vi "test_libssh2_channel_handle_extended_data2.vi"() -> ()   [LabVIEW 2013, in "libssh2_integration_tests.lvlib"]
uses:
  libssh2_integration_tests.lvlib
  <vilib>/addons/_JKI Toolkits/Caraya/classes/Test/Test.lvclass
  support/support.lvlib
  libssh2/libssh2.lvlib
  <vilib>/addons/_JKI Toolkits/Caraya/classes/Assert/Assert.lvclass
panel:
  out "error out":errorcluster
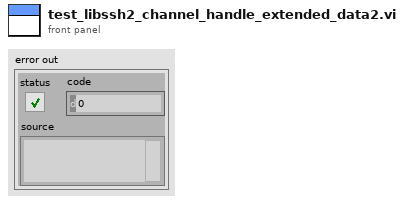
[diagram p1: front panel]
types:
  T1 = cluster{"mode":i32, "stdin":string, "stdout":string, "stderr":string}[]
  T2 = typedef "libssh2.lvlib/Session Refnum.ctl" = refnum<k1>
  T3 = typedef "libssh2.lvlib/Channel Refnum.ctl" = refnum<k1>
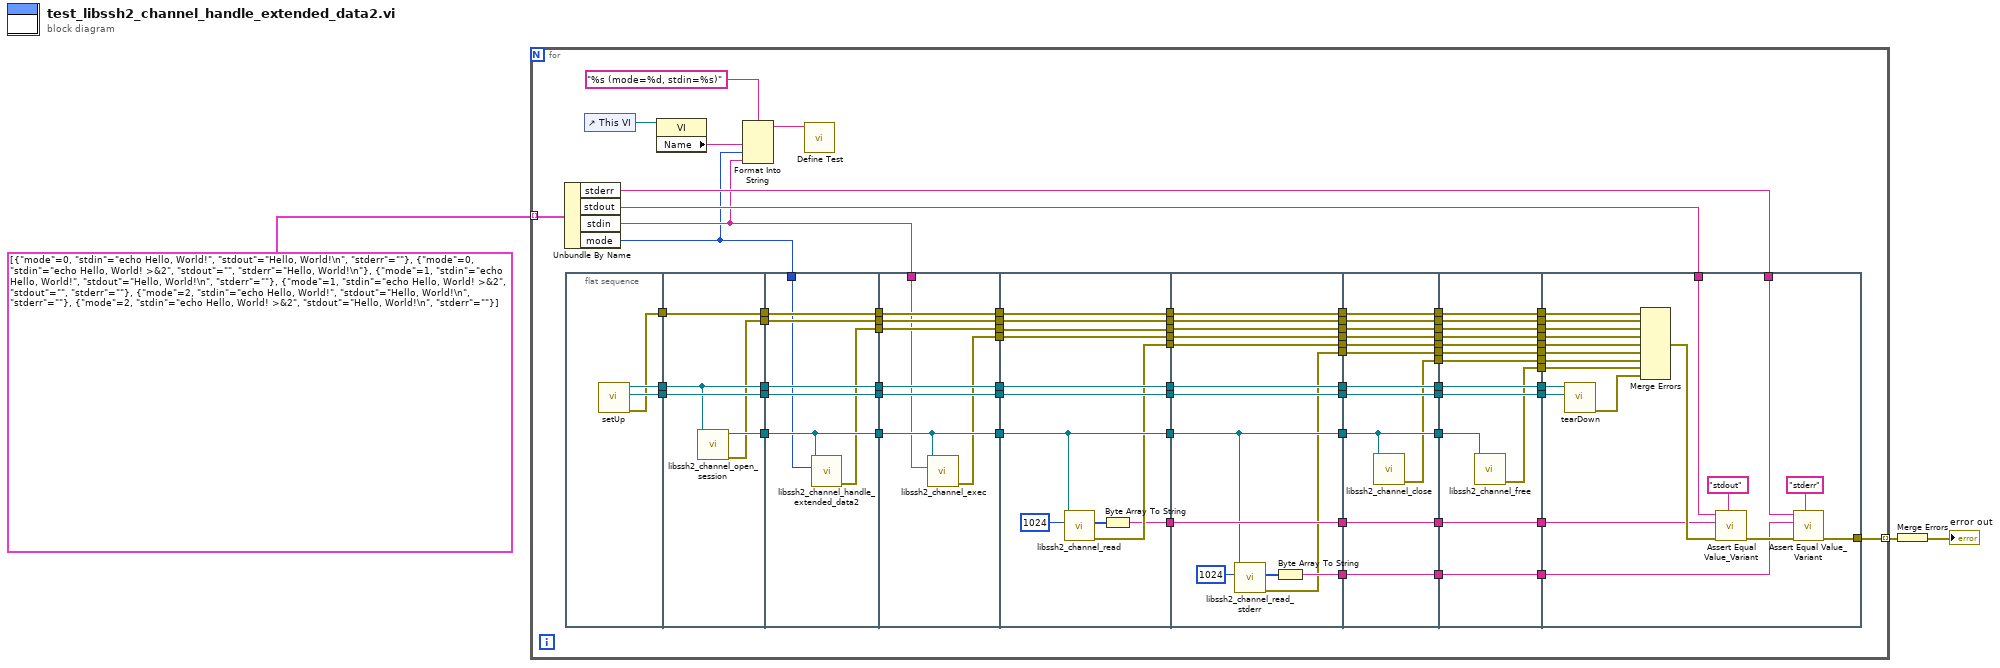
[diagram p0: block diagram]
diagram:
  n1 = for {
    tunnel: T1 [{"mode"=0, "stdin"="echo Hello, World!", "stdout"="Hello, World!\n", "stderr"=""}, {"mode"=0, "stdin"="echo Hello, World! >&2", "stdout"="", "stderr"="Hello, World!\n"}, {"mode"=1, "stdin"="echo Hello, World!", "stdout"="Hello, World!\n", "stderr"=""}, {"mode"=1, "stdin"="echo Hello, World! >&2", "stdout"="", "stderr"=""}, {"mode"=2, "stdin"="echo Hello, World!", "stdout"="Hello, World!\n", "stderr"=""}, {"mode"=2, "stdin"="echo Hello, World! >&2", "stdout"="Hello, World!\n", "stderr"=""}] -> [w35] mode=indexing
    tunnel: [w36] -> w2 mode=indexing
    n2 = Unbundle By Name(w35) -> ("stderr"=w10:string, "stdout"=w47:string, "stdin"=w5:string, "mode"=w4:i32)
    n3 = flat-sequence {
      tunnel: [w81] -> w78
      tunnel: [w80] -> w77
      tunnel: [w79] -> w76
      tunnel: w78 -> [w85]
      tunnel: w77 -> [w86]
      tunnel: [w85] -> w75
      tunnel: [w86] -> w74
      tunnel: [w84] -> w73
      tunnel: w76 -> [w83]
      tunnel: [w83] -> w72
      tunnel: [w82] -> w71
      tunnel: w75 -> [w93]
      tunnel: [w93] -> w70
      tunnel: w74 -> [w92]
      tunnel: [w92] -> w69
      tunnel: w73 -> [w89]
      tunnel: [w89] -> w68
      tunnel: w72 -> [w91]
      tunnel: [w91] -> w67
      tunnel: w71 -> [w90]
      tunnel: [w90] -> w66
      tunnel: w4 -> [w88]
      tunnel: [w87] -> w50
      tunnel: w70 -> [w101]
      tunnel: [w101] -> w65
      tunnel: w69 -> [w100]
      tunnel: [w100] -> w64
      tunnel: w68 -> [w98]
      tunnel: [w98] -> w63
      tunnel: w67 -> [w99]
      tunnel: [w99] -> w62
      tunnel: w66 -> [w97]
      tunnel: [w97] -> w61
      tunnel: [w96] -> w60
      tunnel: w50 -> [w95]
      tunnel: [w95] -> w49
      tunnel: w5 -> [w94]
      tunnel: w65 -> [w112]
      tunnel: [w112] -> w34
      tunnel: w64 -> [w111]
      tunnel: [w111] -> w32
      tunnel: w63 -> [w105]
      tunnel: [w105] -> w30
      tunnel: w62 -> [w110]
      tunnel: [w110] -> w28
      tunnel: w61 -> [w109]
      tunnel: [w109] -> w26
      tunnel: w60 -> [w108]
      tunnel: [w108] -> w24
      tunnel: [w104] -> w22
      tunnel: w49 -> [w107]
      tunnel: [w107] -> w20
      tunnel: [w102] -> w18
      tunnel: w34 -> [w125]
      tunnel: [w125] -> w33
      tunnel: w32 -> [w124]
      tunnel: [w124] -> w31
      tunnel: w30 -> [w117]
      tunnel: [w117] -> w29
      tunnel: w28 -> [w123]
      tunnel: [w123] -> w27
      tunnel: w26 -> [w122]
      tunnel: [w122] -> w25
      tunnel: w24 -> [w121]
      tunnel: [w121] -> w23
      tunnel: w22 -> [w120]
      tunnel: [w120] -> w21
      tunnel: w20 -> [w119]
      tunnel: [w119] -> w19
      tunnel: w18 -> [w118]
      tunnel: [w118] -> w17
      tunnel: [w114] -> w14
      tunnel: [w113] -> w13
      tunnel: w33 -> [w137]
      tunnel: w31 -> [w136]
      tunnel: w29 -> [w135]
      tunnel: [w137] -> w46
      tunnel: [w136] -> w45
      tunnel: [w135] -> w44
      tunnel: [w134] -> w43
      tunnel: w27 -> [w133]
      tunnel: [w133] -> w42
      tunnel: w25 -> [w132]
      tunnel: [w132] -> w41
      tunnel: w23 -> [w131]
      tunnel: [w131] -> w40
      tunnel: w21 -> [w130]
      tunnel: [w130] -> w39
      tunnel: w19 -> [w129]
      tunnel: [w129] -> w37
      tunnel: [w128] -> w38
      tunnel: w17 -> [w128]
      tunnel: [w127] -> w15
      tunnel: w14 -> [w127]
      tunnel: w13 -> [w126]
      tunnel: [w126] -> w12
      tunnel: w46 -> [w150]
      tunnel: w45 -> [w149]
      tunnel: w44 -> [w148]
      tunnel: [w150] -> w59
      tunnel: [w149] -> w58
      tunnel: [w147] -> w57
      tunnel: w43 -> [w146]
      tunnel: [w146] -> w56
      tunnel: w42 -> [w145]
      tunnel: [w145] -> w55
      tunnel: w41 -> [w144]
      tunnel: [w144] -> w54
      tunnel: w40 -> [w143]
      tunnel: [w143] -> w53
      tunnel: w39 -> [w142]
      tunnel: [w142] -> w52
      tunnel: [w141] -> w51
      tunnel: w38 -> [w141]
      tunnel: w37 -> [w140]
      tunnel: [w140] -> w48
      tunnel: [w139] -> w16
      tunnel: w15 -> [w139]
      tunnel: w12 -> [w138]
      tunnel: [w138] -> w11
      tunnel: w59 -> [w170]
      tunnel: w58 -> [w169]
      tunnel: [w154] -> w36
      tunnel: w57 -> [w167]
      tunnel: w56 -> [w166]
      tunnel: w55 -> [w165]
      tunnel: w54 -> [w163]
      tunnel: w53 -> [w162]
      tunnel: w52 -> [w161]
      tunnel: w51 -> [w160]
      tunnel: w48 -> [w159]
      tunnel: w47 -> [w158]
      tunnel: w16 -> [w151]
      tunnel: w11 -> [w156]
      tunnel: w10 -> [w152]
      frame #0 {
        n4 = call "setUp.vi"() -> ("error out"=w79:errorcluster, "connection ID"=w80:refnum<k5>, "session"=w81:T2)  [unwired: 9 in]
      }
      frame #1 {
        n5 = call "libssh2_channel_open_session.vi"("session"=w85) -> ("error out"=w82:errorcluster, "channel"=w84:T3)  [unwired: 9 in]
      }
      frame #2 {
        n6 = call "libssh2_channel_handle_extended_data2.vi"("mode (normal)"=w88, "channel"=w89) -> ("error out"=w87:errorcluster)  [unwired: 9 in]
      }
      frame #3 {
        n7 = call "libssh2_channel_exec.vi"("command"=w94, "channel"=w98) -> ("error out"=w96:errorcluster)  [unwired: 9 in]
      }
      frame #4 {
        n8 = call "libssh2_channel_read.vi"("buffer length"=1024, "channel"=w105) -> ("error out"=w104:errorcluster, "buffer"=w103:u8[])  [unwired: 8 in]
        n9 = Byte Array To String(unsigned byte array=w103) -> (string=w102:string)
      }
      frame #5 {
        n10 = call "libssh2_channel_read_stderr.vi"("buffer length"=1024, "channel"=w117) -> ("error out"=w113:errorcluster, "buffer"=w115:u8[])  [unwired: 8 in]
        n11 = Byte Array To String(unsigned byte array=w115) -> (string=w114:string)
      }
      frame #6 {
        n12 = call "libssh2_channel_close.vi"("channel"=w135) -> ("error out"=w134:errorcluster)  [unwired: 10 in]
      }
      frame #7 {
        n13 = call "libssh2_channel_free.vi"("channel"=w148) -> ("error out"=w147:errorcluster)  [unwired: 10 in]
      }
      frame #8 {
        n14 = call "tearDown.vi"("connection ID"=w169, "session"=w170) -> ("error out"=w168:errorcluster)  [unwired: 9 in]
        n15 = Merge Errors(w165, w163, w159, w162, w161, w156, w166, w167, w168) -> (w164:errorcluster)
        n16 = call <vilib>:"Assert Equal Value_Variant.vi"("Label"="stdout", "error in (no error)"=w164, "Y"=w160, "X"=w158) -> ("error out"=w155:errorcluster)  [unwired: 6 in, 1 out]
        n17 = call <vilib>:"Assert Equal Value_Variant.vi"("Label"="stderr", "error in (no error)"=w155, "Y"=w151, "X"=w152) -> ("error out"=w154:errorcluster)  [unwired: 6 in, 1 out]
      }
    }
    n18 = control-ref of="This VI"() -> (w9:refnum<vi>)
    n19 = property class="VI"(reference=w9) -> ("Name"=w8:string)  [unwired: 1 in, 2 out]
    n20 = Format Into String(format string="%s (mode=%d, stdin=%s)", w8, w4, w5) -> (resulting string=w6:string)  [unwired: 2 in, 1 out]
    n21 = call <vilib>:"Define Test.vi"("Label (VI Title)"=w6) -> ()  [unwired: 9 in, 2 out]
  }
  n22 = Merge Errors(w2) -> (→"error out":errorcluster)
